vi "Write TDMS with Converted RawDataQ ScanData.vi"(6 "dt(s)":dbl, 7 "Enable TDMS Write":bool, 8 "error in (no error)":errorcluster, 9 "DAQ RawData Q":T1, 10 "tdms ref":refnum<k34>, 11 "LogEngine in":refnum<class "LogEngine.lvclass">) -> (0 "error out":errorcluster, 3 "LogEngine out":refnum<class "LogEngine.lvclass">)   [LabVIEW 2017, in "LogEngine.lvclass"]
doc: "Developed by Kevin Thompson\nkevin@thompsonengineering.net\n\nCopyright 2018-2020\nThompson Engineering, LLC"
uses:
  LogEngine.lvclass
  Support/DataQueues/DataTypes/Analog DataSet MultiRow & ChanNames--QRef.ctl
  Support/DataQueues/DataTypes/Analog DataSet MultiRow & ChanNames--cluster.ctl
  Support/DataQueues/DataQueues.lvclass
panel:
  out "DAQ Scan Wfm[]":waveform(dbl)[](array[waveform])
  # "This array from EACH DAQ RawData Q element.\nIt is updated as each element is converted."
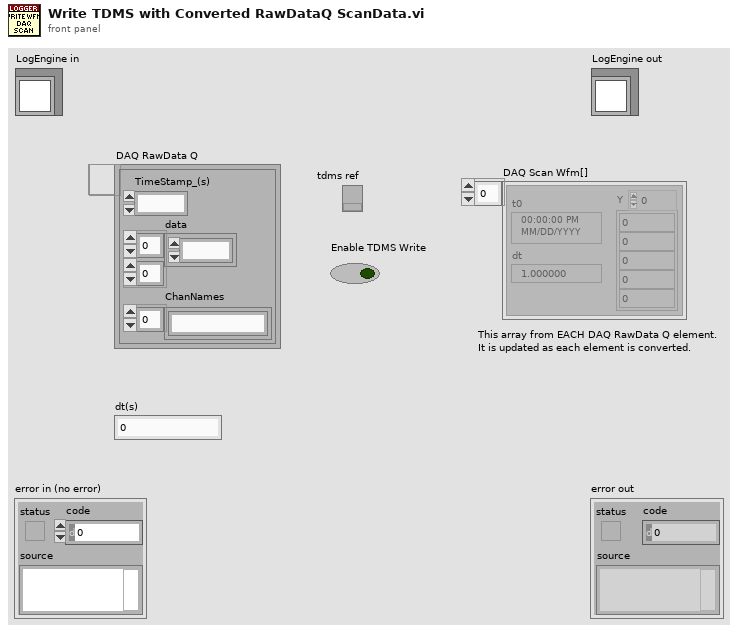
[diagram p1: front panel]
types:
  T1 = typedef "DataQueues.lvclass/Analog DataSet MultiRow & ChanNames--QRef.ctl" = refnum<queue>
  T2 = typedef "DataQueues.lvclass/Analog DataSet MultiRow & ChanNames--cluster.ctl" = cluster{"TimeStamp_(s)":dbl, "data":dbl[][], "ChanNames":string[]}
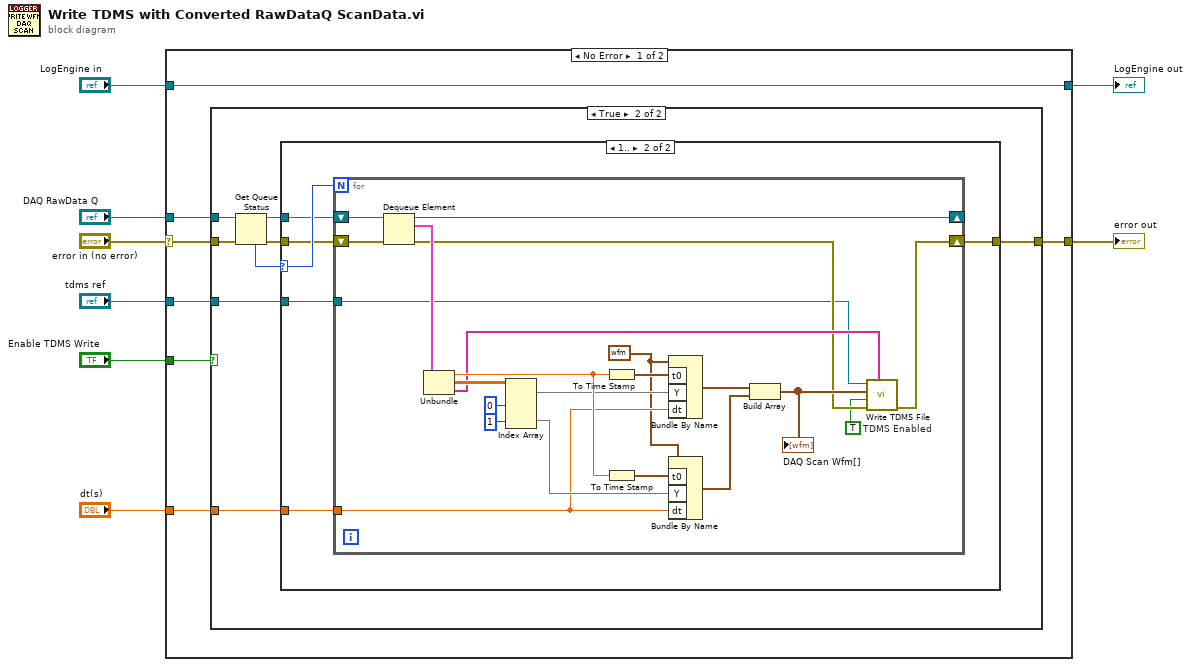
[diagram p0: block diagram]
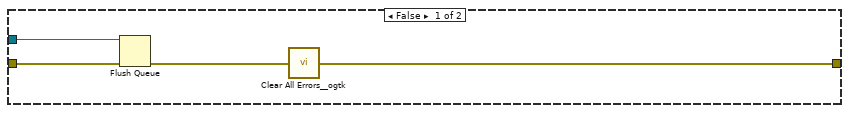
[diagram p2: hidden frame]
diagram:
  n1 = case shown="No Error" "error in (no error)" {
    selector: "error in (no error)" -> [w13 w57]
    tunnel: [w15 w58] -> w6
    tunnel: "LogEngine in" -> [w15 w58]
    tunnel: "DAQ RawData Q" -> [w14 _]
    tunnel: "dt(s)" -> [w12 _]
    tunnel: "tdms ref" -> [w11 _]
    tunnel: "Enable TDMS Write" -> [w9 _]
    tunnel: [w10 w57] -> w1
    frame No Error {
      n2 = case shown="True" w9 {
        tunnel: w14 -> [w19 w27]
        tunnel: w13 -> [w18 w24]
        tunnel: w12 -> [_ w22]
        tunnel: w11 -> [_ w21]
        tunnel: [w16 w20] -> w10
        frame False {
          n3 = Flush Queue(queue=w19, error in (no error)=w18) -> (error out=w17:errorcluster)  [unwired: 2 out]
          n4 = call <userlib>:"Clear All Errors__ogtk.vi"("Error In"=w17) -> ("Error Out"=w16:errorcluster)  [unwired: 3 in]
        }
        frame True {
          n5 = Get Queue Status(queue=w27, error in (no error)=w24) -> (queue out=w25:T1, error out=w23:errorcluster, # elements in queue=w26:i32)  [unwired: 1 in, 5 out]
          n6 = case shown="1.." w26 {
            selector: w26 -> [_ w34]
            tunnel: w25 -> [_ w33]
            tunnel: w23 -> [w28 w32]
            tunnel: w22 -> [_ w31]
            tunnel: w21 -> [_ w30]
            tunnel: [w28 w29] -> w20
            frame ..0 {
            }
            frame 1.. {
              n7 = for {
                N: w34 -> [_]
                shift-right: [w37] -> w29
                shift-left: w32 -> [w55]
                shift-right: [w54] -> _
                shift-left: w33 -> [w56]
                tunnel: w31 -> [w44]
                tunnel: w30 -> [w35]
                w36 = TRUE  # TDMS Enabled
                w39 = waveform(dbl) {"t0"=timestamp(0 s since 1904-01-01), "dt"=1.0, "Y"=[]} ("waveform")
                n8 = Dequeue Element(queue=w56, error in (no error)=w55) -> (queue out=w54:T1, element=w53:T2, error out=w38:errorcluster)  [unwired: 1 in, 1 out]
                n9 = Unbundle(w53) -> ("TimeStamp_(s)"=w50:dbl, "data"=w49:dbl[][], "ChanNames"=w40:string[])
                n10 = Index Array(array=w49, index (row) #1=0 ("index (row)"), index (row) #2=1 ("index (row)")) -> (element #1=w46:dbl[], element #2=w45:dbl[])  [unwired: 2 in]
                n11 = To Time Stamp(1:w50) -> (0:w52:timestamp)
                n12 = To Time Stamp(1:w50) -> (0:w51:timestamp)
                n13 = Bundle By Name(cluster=w39, "t0"=w52, "Y"=w46, "dt"=w44) -> (w43:waveform(dbl))
                n14 = Bundle By Name(cluster=w39, "t0"=w51, "Y"=w45, "dt"=w44) -> (w42:waveform(dbl))
                n15 = Build Array(w43, w42) -> (w41:waveform(dbl)[])
                "DAQ Scan Wfm[]" <- w41
                n16 = call "Write TDMS File.vi"("channel name(s)"=w40, "error in (no error)"=w38, "TDMS Enabled"=w36, "Wfm data (NChanNSamp)"=w41, "tdms ref"=w35) -> ("error out"=w37:errorcluster)  [unwired: 5 in, 1 out]
              }
            }
          }
        }
      }
    }
    frame Error {
    }
  }
  "error out" <- w1
  "LogEngine out" <- w6
